vi "Fault Id 2 String.vi"(9 "Add LBCB Type":bool, 10 "Fault Id In":T1={"Fault Type"=enum."Force", "LBCB Number"=enum."LBCB2", "Index"=3, "Space Type"=enum."Cartesian"}) -> (2 "String":string=" Cartesian Force Cartesian Moment Mx (lb*in)")   [LabVIEW 2013]
uses:
  Fault Id.ctl
  Fault Type.ctl
  Data Access Objects/Metadata/LBCB Number.ctl
  Space Type.ctl
panel:
  in  "Actuators":string[](array[string])=[" X1", " X2", " Y1", " Z1", " Z2", " Z3"]
  in  "Cartesian\nForce":string[](array[string])=["Fx", "Fy", "Fz", "Mx", "My", "Mz"]
  in  "Cartesian \nDisplacement":string[](array[string])=["Dx", "Dy", "Dz", " Rx (rad)", " Ry (rad)", " Rz (rad)"]
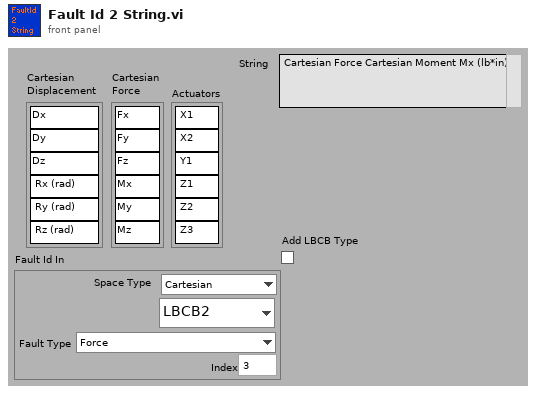
[diagram p1: front panel]
types:
  T1 = typedef "Fault Id.ctl" = cluster{"Fault Type":T2, "LBCB Number":T3, "Index":u32, "Space Type":T4}
  T2 = typedef "Fault Type.ctl" = enum16{"None", "Command", "Displacement", "Force", "Increment"}
  T3 = typedef "LBCB Number.ctl" = enum16{"LBCB1", "LBCB2"}
  T4 = typedef "Space Type.ctl" = enum16{"Actuator", "Cartesian"}
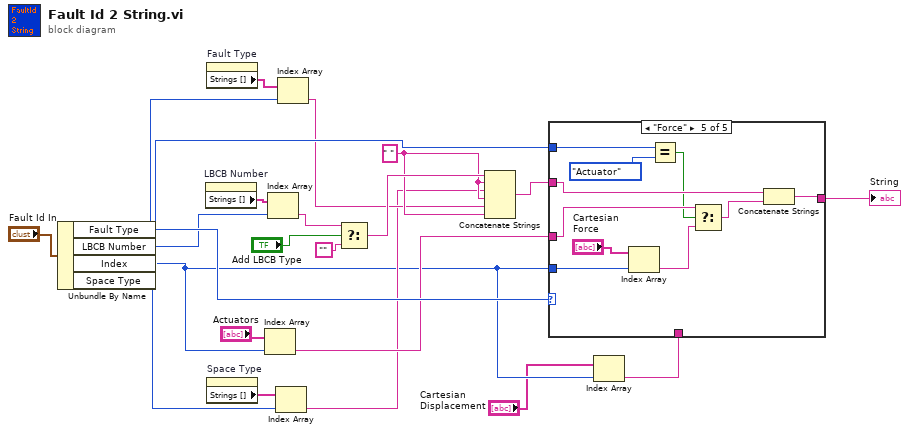
[diagram p0: block diagram]
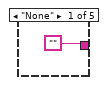
[diagram p2: hidden frame]
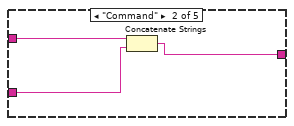
[diagram p3: hidden frame]
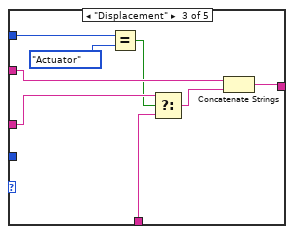
[diagram p4: hidden frame]
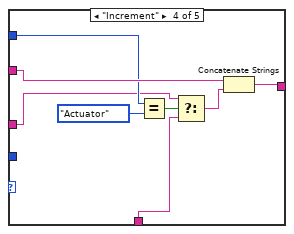
[diagram p5: hidden frame]
diagram:
  w7 = " "
  n1 = Unbundle By Name("Fault Id In") -> ("Fault Type"=w19:T2, "LBCB Number"=w17:T3, "Index"=w3:u32, "Space Type"=w6:T4)
  n2 = property on="LBCB Number" class="Enum (strict)"() -> ("Strings []"=w18:string[])  [unwired: 2 in, 2 out]
  n3 = property on="Fault Type" class="Enum (strict)"() -> ("Strings []"=w20:string[])  [unwired: 2 in, 2 out]
  n4 = property on="Space Type" class="Enum (strict)"() -> ("Strings []"=w12:string[])  [unwired: 2 in, 2 out]
  n5 = Index Array(array="Actuators", index=w3) -> (element=w9:string)
  n6 = Index Array(array=w18, index=w17) -> (element=w16:string)
  n7 = Index Array(array=w12, index=w6) -> (element=w4:string)
  n8 = Index Array(array=w20, index=w19) -> (element=w5:string)
  n9 = Select(t=w16, s="Add LBCB Type", f="") -> (s? t:f=w11:string)
  n10 = Concatenate Strings(w11, w7, w4, w7, w5, w7) -> (w10:string)
  n11 = Index Array(array="Cartesian \nDisplacement", index=w3) -> (element=w1:string)
  n12 = case shown="\"Force\"" w19 {
    tunnel: w10 -> [_ w25 w33 w41 w50]
    tunnel: w9 -> [_ w24 w31 w35 w47]
    tunnel: ["" w23 w27 w40 w43] -> w8
    tunnel: w3 -> [_ _ _ _ w51]
    tunnel: w6 -> [_ _ w30 w38 w46]
    tunnel: w1 -> [_ _ w26 w34 _]
    frame "None" {
    }
    frame "Command" {
      n13 = Concatenate Strings(w25, w24) -> (w23:string)
    }
    frame "Displacement" {
      n14 = Equal?(x=w30, y=Space_Type."Actuator") -> (x = y?=w29:bool)
      n15 = Select(t=w31, s=w29, f=w26) -> (s? t:f=w32:string)
      n16 = Concatenate Strings(w33, w32) -> (w27:string)
    }
    frame "Increment" {
      n17 = Equal?(x=w38, y=Space_Type."Actuator") -> (x = y?=w39:bool)
      n18 = Select(t=w35, s=w39, f=w34) -> (s? t:f=w36:string)
      n19 = Concatenate Strings(w41, w36) -> (w40:string)
    }
    frame "Force" {
      n20 = Index Array(array="Cartesian\nForce", index=w51) -> (element=w48:string)
      n21 = Equal?(x=w46, y=Space_Type."Actuator") -> (x = y?=w45:bool)
      n22 = Select(t=w47, s=w45, f=w48) -> (s? t:f=w49:string)
      n23 = Concatenate Strings(w50, w49) -> (w43:string)
    }
  }
  "String" <- w8
